vi "Numbers.vi"(0 "Numbers in":refnum<class "Numbers.lvclass">, 5 "Number1":dbl, 7 "Number2":dbl, 9 "CalculationWanted":string, 11 "error in (no error)":errorcluster) -> (4 "Numbers out":refnum<class "Numbers.lvclass">, 15 "error out":errorcluster)   [LabVIEW 2017, in "Numbers.lvclass"]
uses:
  Numbers.lvclass
  Numbers.lvclass/Numbers.ctl
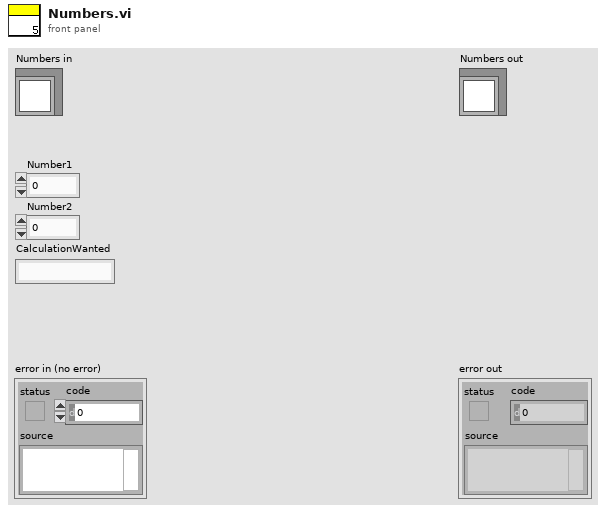
[diagram p1: front panel]
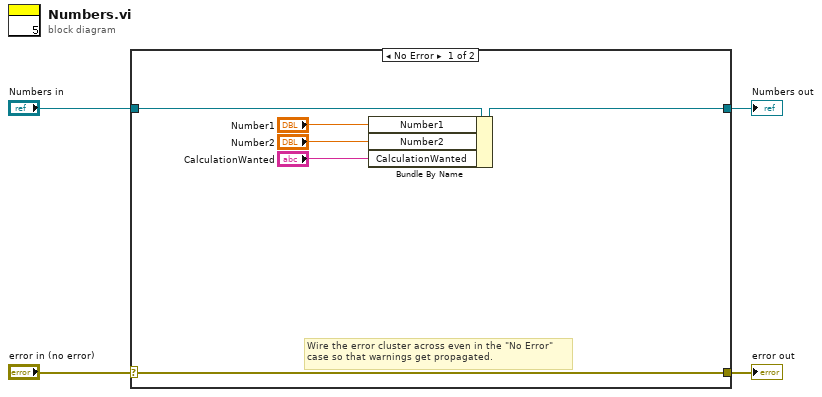
[diagram p0: block diagram]
diagram:
  n1 = case shown="No Error" "error in (no error)" {
    selector: "error in (no error)" -> [w9 w12]
    tunnel: [w9 w12] -> w3
    tunnel: [w8 w11] -> w1
    tunnel: "Numbers in" -> [w10 w11]
    frame No Error {
      # "Wire the error cluster across even in the \"No Error\"\ncase so that warnings get propagated."
      n2 = Bundle By Name(cluster=w10, "Number1"="Number1", "Number2"="Number2", "CalculationWanted"="CalculationWanted") -> (w8:refnum<class "Numbers.lvclass">)
    }
    frame Error {
    }
  }
  "error out" <- w3
  "Numbers out" <- w1
